vi "FFT1D_Top.vi"() -> ()   [LabVIEW 2020]
doc: "This benchmark is designed to demonstrate execution performance improvement when executing FFT and IFFT operations on a GPU."
uses:
  <vilib>/Ngene/CuLab - GPU Accelerated Toolkit/Toolkit/CuLab.lvlib
  <vilib>/Analysis/NI_AALBase.lvlib
  <vilib>/Analysis/1siggen.llb/Ramp Pattern by Delta.vi
  <vilib>/Analysis/baseanly.llb/Mean (DBL).vi
  <vilib>/Utility/file.llb/Read Delimited Spreadsheet (DBL).vi
panel:
  in  "CPU Iteration":i32=3
  out "CuLab Mean Performance Gain":dbl[](array[numeric])=[1.0, 15.094286206296445, 1.9171194489701426] format="%#.2g"
  out "Releative Exec Time vs CuLab (smaller is better)":cluster{i32[], "all rows":dbl[]}[](graph)=[{[1024, 2048, 4096, 8192, 16384, 32768, 65536, 131072, 262144, 524288, 1048576, 2097152, 4194304, 8388608, 16777216, 33554432, 67108864], "all rows"=[1.0, 1.0, 1.0, 1.0, 1.0, 1.0, 1.0, 1.0, 1.0, 1.0, 1.0, 1.0, 1.0, 1.0, 1.0, 1.0, 1.0]}, {[1024, 2048, 4096, 8192, 16384, 32768, 65536, 131072, 262144, 524288, 1048576, 2097152, 4194304, 8388608, 16777216, 33554432, 67108864], "all rows"=[0.28326995573146957, 0.4744744711527261, 0.7891705062605822, 1.4352640500932945, 2.2928719150994206, 4.083834886813619, 5.835875710159926, 6.6859728440246355, 10.169029556785343, 17.39591860482113, 20.72043338307738, 23.170923254755827, 25.23511813570062, 27.50988798473057, 32.05325123298233, 39.76444417476331, 38.70312484008737]}, {[1024, 2048, 4096, 8192, 16384, 32768, 65536, 131072, 262144, 524288, 1048576, 2097152, 4194304, 8388608, 16777216, 33554432, 67108864], "all rows"=[3.88973381481515, 3.138138155703473, 2.4792626543916514, 1.9574105485466562, 1.400826453766223, 1.3662940596991726, 1.237853108084698, 1.4708898928363592, 1.5527156554884731, 1.6561805635204403, 1.6882342202321916, 1.7257126953492796, 1.8068059027564272, 1.8125554033459044, 1.7960561428250041, 1.8055172134477608, 1.8068441476835568]}]
  in  "CuPy CSV":path=path "D:/Ngene/GitHub/culab_examples/Benchmarks/CuPy/results/GeForce_RTX_2080_Ti/FFT1D_CuPy.csv"
  out "Execution Time":cluster{i32[], "all rows":dbl[]}[](graph)=[{[1024, 2048, 4096, 8192, 16384, 32768, 65536, 131072, 262144, 524288, 1048576, 2097152, 4194304, 8388608, 16777216, 33554432, 67108864], "all rows"=[2.6300000172341242e-05, 3.329999981360743e-05, 4.340000032243552e-05, 5.870000040886225e-05, 9.679999948275508e-05, 0.00011630000062723411, 0.00017699999989417847, 0.00033150000035675475, 0.0005007999998269952, 0.0008551000000807107, 0.0016428999997515348, 0.0032342000004064175, 0.006200499999977183, 0.012408999999934167, 0.025107399999797053, 0.04933649999929912, 0.097768200000246]}, {[1024, 2048, 4096, 8192, 16384, 32768, 65536, 131072, 262144, 524288, 1048576, 2097152, 4194304, 8388608, 16777216, 33554432, 67108864], "all rows"=[7.449999884556746e-06, 1.5799999800947262e-05, 3.4250000226165866e-05, 8.425000032730168e-05, 0.0002219500001956476, 0.0004749499998979445, 0.0010329500000807457, 0.0022164000001794193, 0.005092650000278809, 0.014875250000386586, 0.03404159999990952, 0.07493939999994836, 0.1564703499998359, 0.3413702000007106, 0.8047738000004756, 1.96183850000034, 3.7839348500001506]}, {[1024, 2048, 4096, 8192, 16384, 32768, 65536, 131072, 262144, 524288, 1048576, 2097152, 4194304, 8388608, 16777216, 33554432, 67108864], "all rows"=[0.0001023, 0.0001045, 0.00010760000000000001, 0.0001149, 0.00013560000000000002, 0.0001589, 0.0002191, 0.00048760000000000003, 0.0007776, 0.0014162, 0.0027736, 0.0055813, 0.0112031, 0.022492, 0.045094300000000004, 0.0890779, 0.1766519]}]
  out "GPU Model":string="NVIDIA GeForce RTX 2080 Ti"
  out "CPU Model":string="Intel(R) Core(TM) i7-8700K"
  in  "GPU Iteration":i32=200
  in  "Size Stop(2^n)":i32=26
  in  "Size Start(2^n)":i32=10
  out "Size":i32[](array[numeric])=[1024, 2048, 4096, 8192, 16384, 32768, 65536, 131072, 262144, 524288, 1048576, 2097152, 4194304, 8388608, 16777216, 33554432, 67108864] format="%.2p"
  # "FFT1D Benchmark"
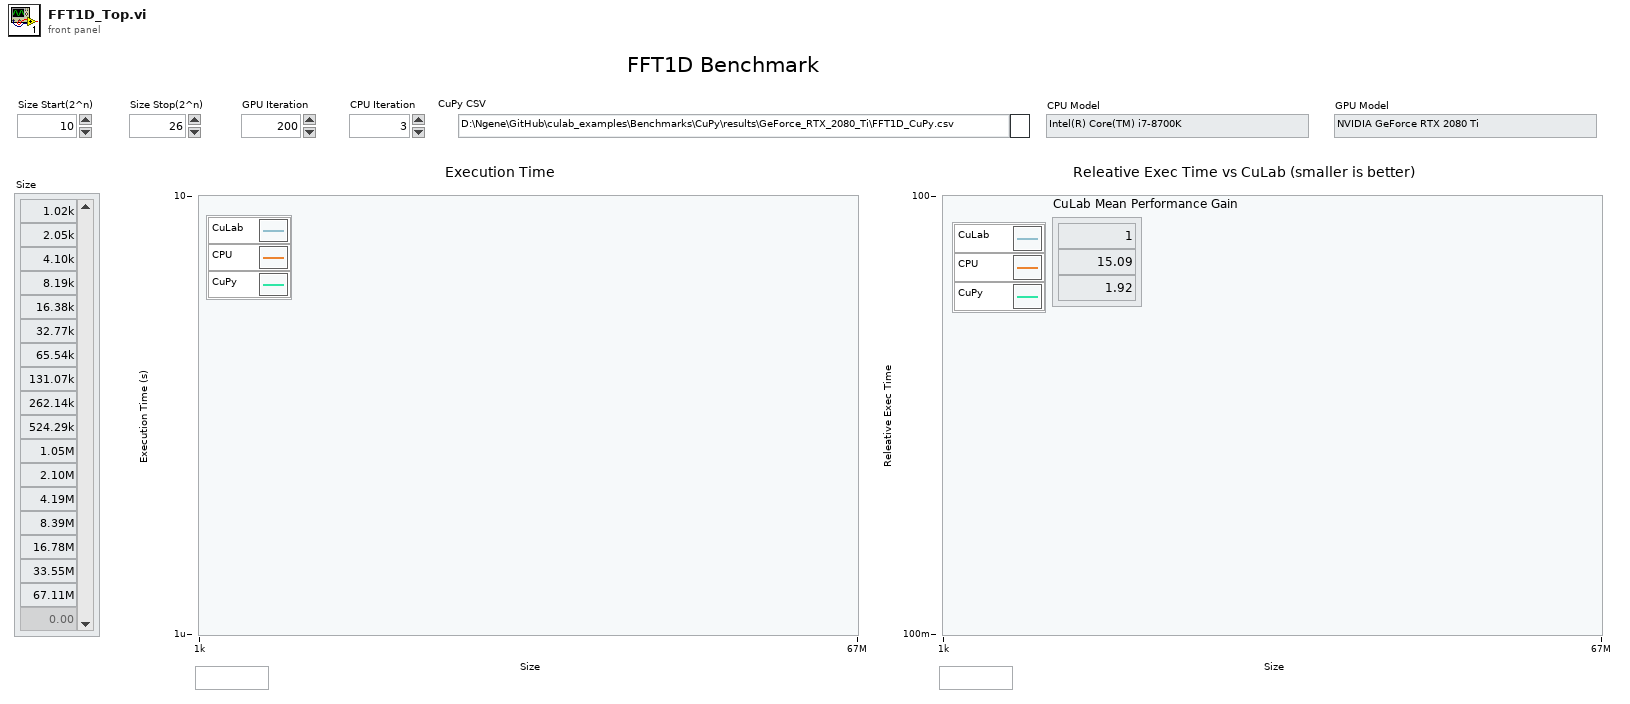
[diagram p1: front panel]
types:
  T1 = typedef "CuLab.lvlib/Properties.ctl" = cluster{"Device ID":i32, "Name":string}
  T2 = typedef "imagedata.ctl" = cluster{"image type":i32, "image depth":i32, "image":u8[], "mask":u8[], "colors":u32[], "Rectangle":cluster{"left":i16, "top":i16, "right":i16, "bottom":i16}}
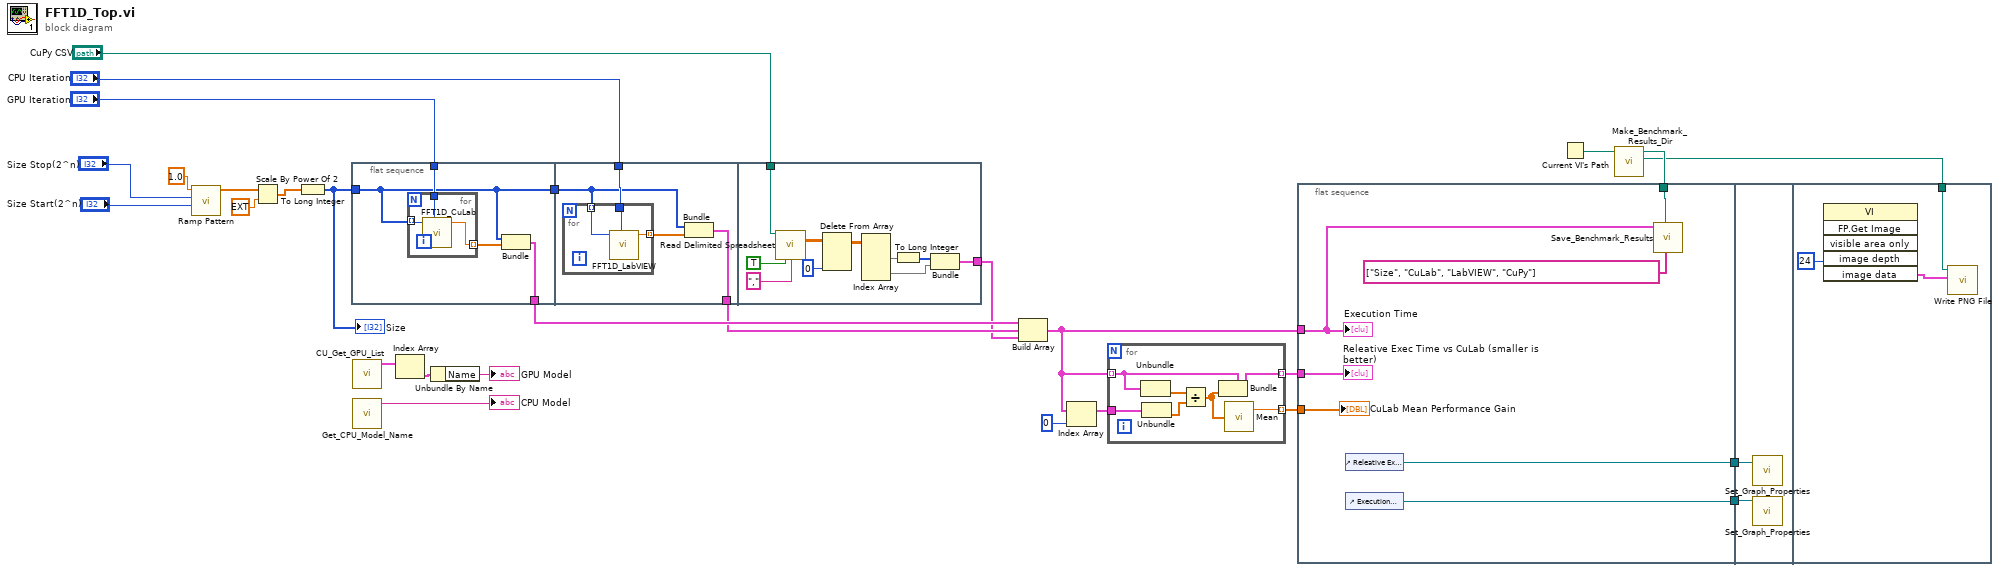
[diagram p0: block diagram]
diagram:
  n1 = call-poly <vilib>:"Ramp Pattern.vi"("start"="Size Start(2^n)", "end"="Size Stop(2^n)", "delta"=1.0) -> ("Ramp Pattern"=w9:dbl[])  [unwired: 6 in, 2 out]
  n2 = Scale By Power Of 2(n=w9, x=ext 1.0) -> (x*2^n=w11:ext[])
  n3 = To Long Integer(number=w11) -> (32bit integer=w8:i32[])
  "Size" <- w8
  n4 = flat-sequence {
    tunnel: [w29] -> w19
    tunnel: [w30] -> w23
    tunnel: w8 -> [w30]
    tunnel: "GPU Iteration" -> [w32]
    tunnel: w23 -> [w37]
    tunnel: "CPU Iteration" -> [w39]
    tunnel: [w36] -> w17
    tunnel: "CuPy CSV" -> [w52]
    tunnel: [w44] -> w15
    frame #0 {
      n5 = for {
        tunnel: w32 -> [w33]
        tunnel: w30 -> [w34] mode=indexing
        tunnel: [w35] -> w31 mode=indexing
        n6 = call "FFT1D_CuLab.vi"("Iteration"=w33, "samples"=w34) -> ("Results(s)"=w35:dbl)  [unwired: 9 in]
      }
      n7 = Bundle(w30, w31) -> (w29:cluster{i32[], dbl[]})  [unwired: 1 in]
    }
    frame #1 {
      n8 = for {
        tunnel: w37 -> [w42] mode=indexing
        tunnel: w39 -> [w40]
        tunnel: [w41] -> w38 mode=indexing
        n9 = call "FFT1D_LabVIEW.vi"("Iteration"=w40, "Samples"=w42) -> ("Results(s)"=w41:dbl)  [unwired: 9 in]
      }
      n10 = Bundle(w37, w38) -> (w36:cluster{i32[], dbl[]})  [unwired: 1 in]
    }
    frame #2 {
      n11 = call-poly <vilib>:"Read Delimited Spreadsheet.vi"("file path (dialog if empty)"=w52, "transpose? (F)"=TRUE, "delimiter (\\t)"="," ("delimiter (\\t)")) -> ("all rows"=w50:dbl[][])  [unwired: 7 in, 5 out]
      n12 = Delete From Array(array=w50, index (col)=0 ("disabled index (col)")) -> (array with subset deleted=w48:dbl[][])  [unwired: 2 in, 1 out]
      n13 = Index Array(array=w48) -> (element #1=w47:dbl[], element #2=w45:dbl[])  [unwired: 4 in]
      n14 = To Long Integer(number=w47) -> (32bit integer=w46:i32[])
      n15 = Bundle(w46, "all rows"=w45) -> (w44:cluster{i32[], "all rows":dbl[]})  [unwired: 1 in]
    }
  }
  n16 = call <vilib>:"CU_Get_GPU_List.vi"() -> ("Devices"=w21:T1[])  [unwired: 10 in, 1 out]
  n17 = call "Get_CPU_Model_Name.vi"() -> ("CPU Model"=→"CPU Model":string)  [unwired: 11 in]
  n18 = Index Array(array=w21) -> (element=w20:T1)  [unwired: 1 in]
  n19 = Unbundle By Name(w20) -> ("Name"=→"GPU Model":string)
  n20 = Build Array(w19, w17, w15) -> (w24:cluster{i32[], "all rows":dbl[]}[])
  n21 = Index Array(array=w24, index=0) -> (element=w28:cluster{i32[], "all rows":dbl[]})
  n22 = for {
    tunnel: w24 -> [w59] mode=indexing
    tunnel: w28 -> [w57]
    tunnel: [w58] -> w26 mode=indexing
    tunnel: [w53] -> w25 mode=indexing
    n23 = Unbundle(w59) -> ("all rows"=w56:dbl[])  [unwired: 1 out]
    n24 = Unbundle(w57) -> ("all rows"=w55:dbl[])  [unwired: 1 out]
    n25 = Divide(x=w56, y=w55) -> (x/y=w54:dbl[])
    n26 = Bundle(cluster=w59, "all rows"=w54) -> (w58:cluster{i32[], "all rows":dbl[]})  [unwired: 1 in]
    n27 = call-poly <vilib>:"Mean.vi"("X"=w54) -> ("mean"=w53:dbl)  [unwired: 1 out]
  }
  n28 = flat-sequence {
    tunnel: w26 -> [w62]
    tunnel: w25 -> [w66]
    tunnel: w24 -> [w63]
    tunnel: w4 -> [w65]
    tunnel: [w61] -> w2
    tunnel: [w60] -> w1
    tunnel: w2 -> [w68]
    tunnel: w1 -> [w67]
    tunnel: w3 -> [w70]
    frame #0 {
      n29 = control-ref of="Releative Exec Time vs CuLab (smaller is better)"() -> (w61:refnum<vi>)
      n30 = control-ref of="Execution Time"() -> (w60:refnum<vi>)
      n31 = call "Save_Benchmark_Results.vi"("Header"=string[] ["Size", "CuLab", "LabVIEW", "CuPy"], "file path (dialog if empty)"=w65, "Execution Time"=w63) -> ()  [unwired: 9 in]
      "Execution Time" <- w63
      "CuLab Mean Performance Gain" <- w66
      "Releative Exec Time vs CuLab (smaller is better)" <- w62
    }
    frame #1 {
      n32 = call "Set_Graph_Properties.vi"("Graph"=w68) -> ()  [unwired: 11 in]
      n33 = call "Set_Graph_Properties.vi"("Graph"=w67) -> ()  [unwired: 11 in]
    }
    frame #2 {
      n34 = invoke class="VI" method="FP.Get Image"("image depth"=24 ("Image Depth")) -> ("image data"=w71:T2)  [unwired: 5 in, 5 out]
      n35 = call <vilib>:"Write PNG File.vi"("image data"=w71, "path to PNG file"=w70) -> ()  [unwired: 8 in, 2 out]
    }
  }
  n36 = Current VI's Path() -> (path=w5:path)
  n37 = call "Make_Benchmark_Results_Dir.vi"("Caller Path"=w5) -> ("Caller FP Image Path"=w3:path, "CSV_File"=w4:path)  [unwired: 9 in]
